vi "CSS811_Main.vi"(8 "error in":errorcluster, 11 "Enum":T1) -> (0 "error out":errorcluster, 2 "CSS811CO2_ppm":u16, 3 "CSS811_VOCppb":u16)   [LabVIEW 2016]
uses:
  CSS811_StateMachine.ctl
  <vilib>/myRIO/Instrument Drivers/Onboard IO/I2C/vis/Configure.vi
  <vilib>/myRIO/Instrument Drivers/Onboard IO/I2C/vis/Write.vi
  <vilib>/myRIO/Instrument Drivers/Onboard IO/I2C/vis/Read.vi
  <vilib>/myRIO/Instrument Drivers/Onboard IO/I2C/vis/Smart Open.vi
  <vilib>/Utility/error.llb/Error Cluster From Error Code.vi
  <vilib>/myRIO/Common/Instrument Driver Framework/myRIO v1.0/I2C/vis/myRIO v1.0 Configure I2C.vi
  <vilib>/myRIO/Common/Instrument Driver Framework/myRIO v1.0/I2C/vis/myRIO v1.0 Write I2C.vi
  <vilib>/myRIO/Common/Instrument Driver Framework/myRIO v1.0/I2C/vis/myRIO v1.0 Read I2C.vi
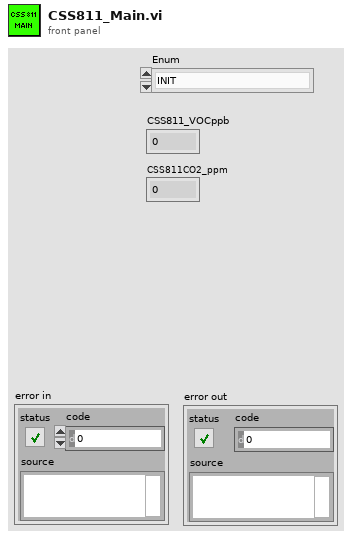
[diagram p1: front panel]
types:
  T1 = typedef "CSS811_StateMachine.ctl" = enum16{"INIT", "CHECK_STATUS", "SET_SENSOR_MODE", "SET_MEASURE_INTERVALL", "GET_SENSOR_DATA", "END", "RESET", "ERROR"}
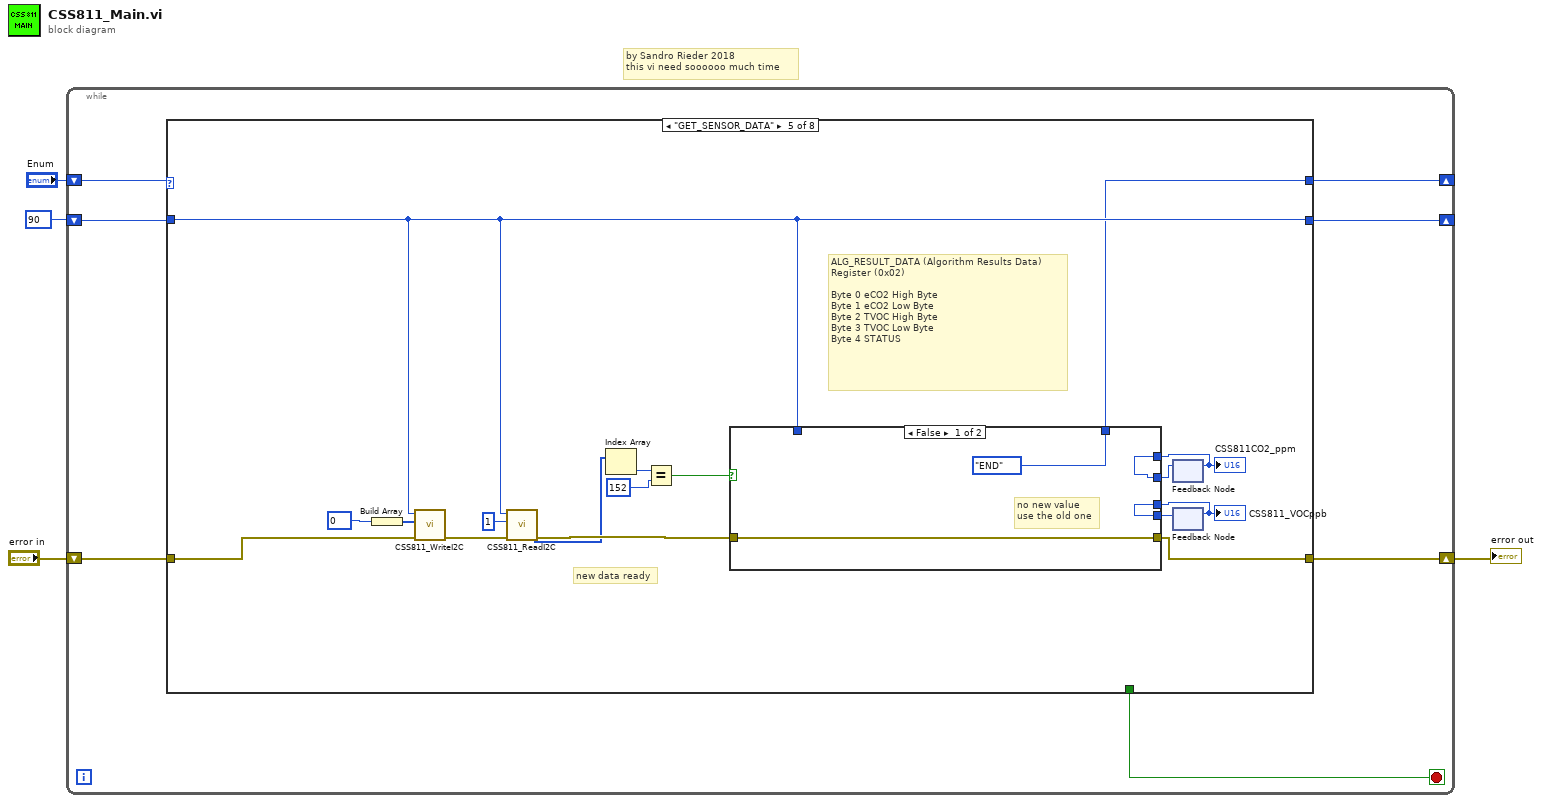
[diagram p0: block diagram]
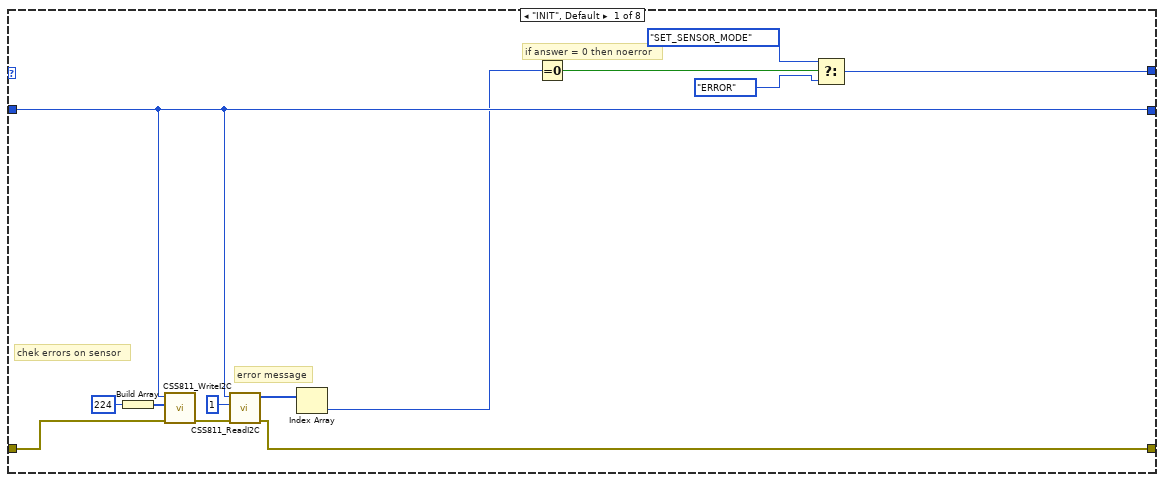
[diagram p2: hidden frame]
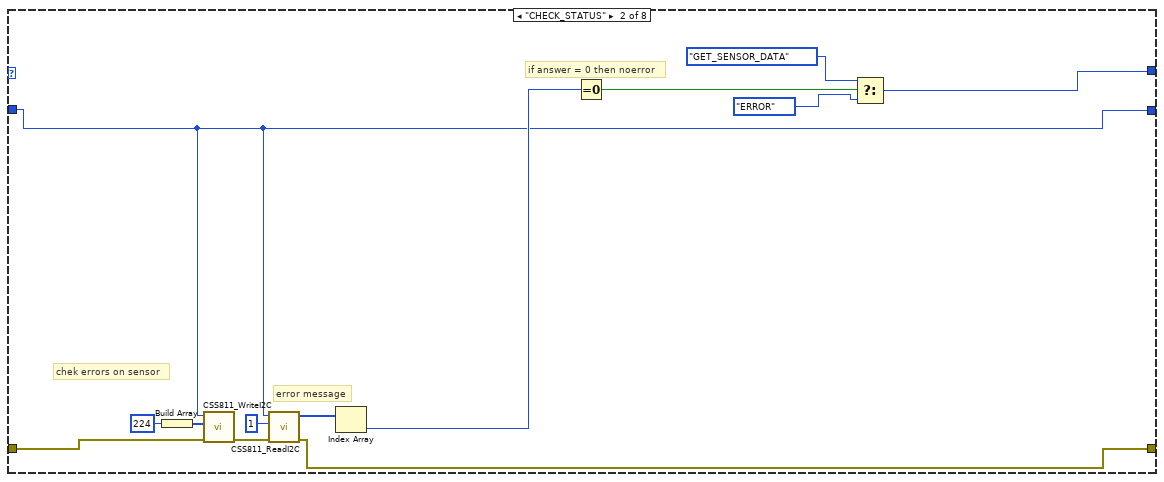
[diagram p3: hidden frame]
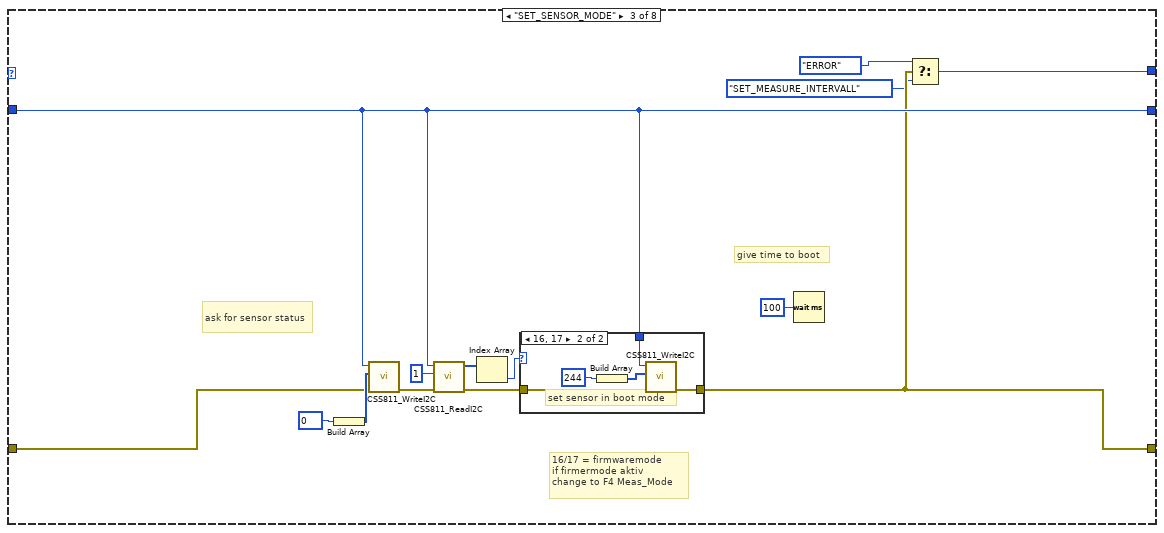
[diagram p4: hidden frame]
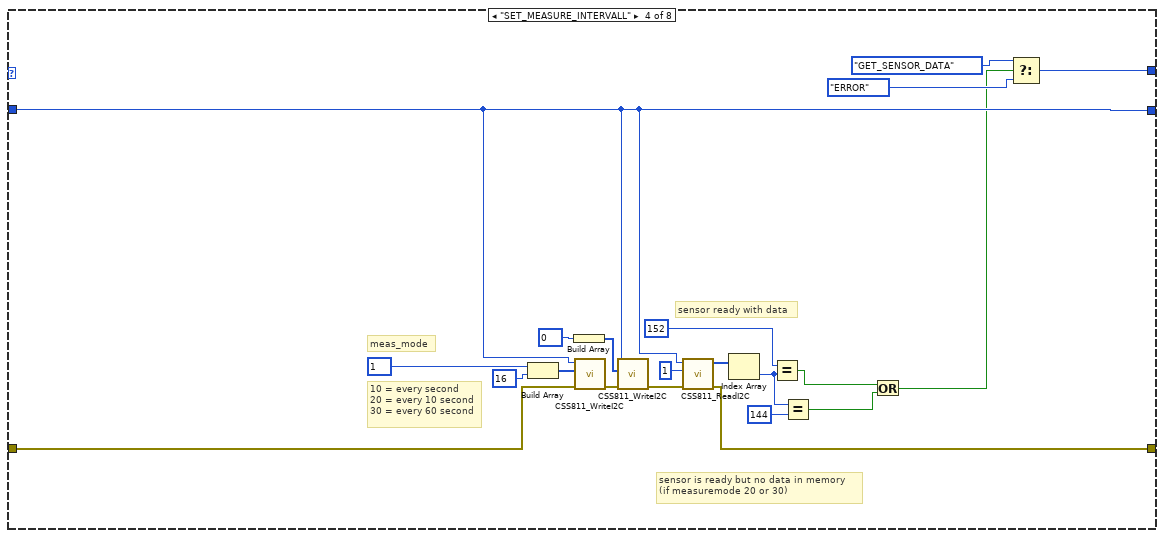
[diagram p6: hidden frame]
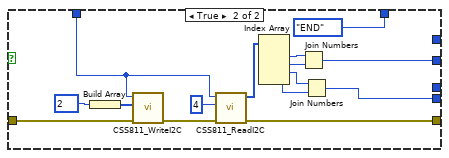
[diagram p7: hidden frame]
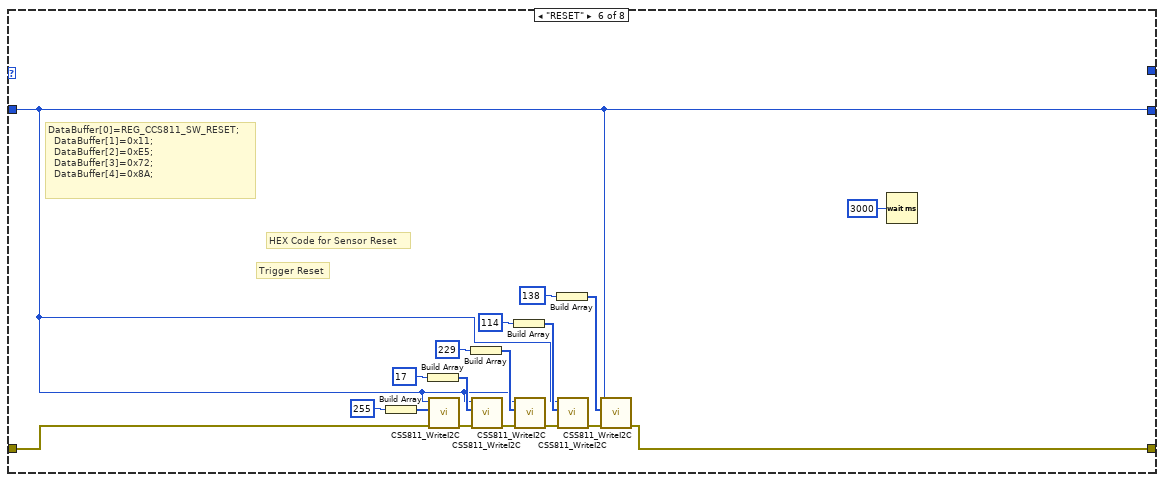
[diagram p8: hidden frame]
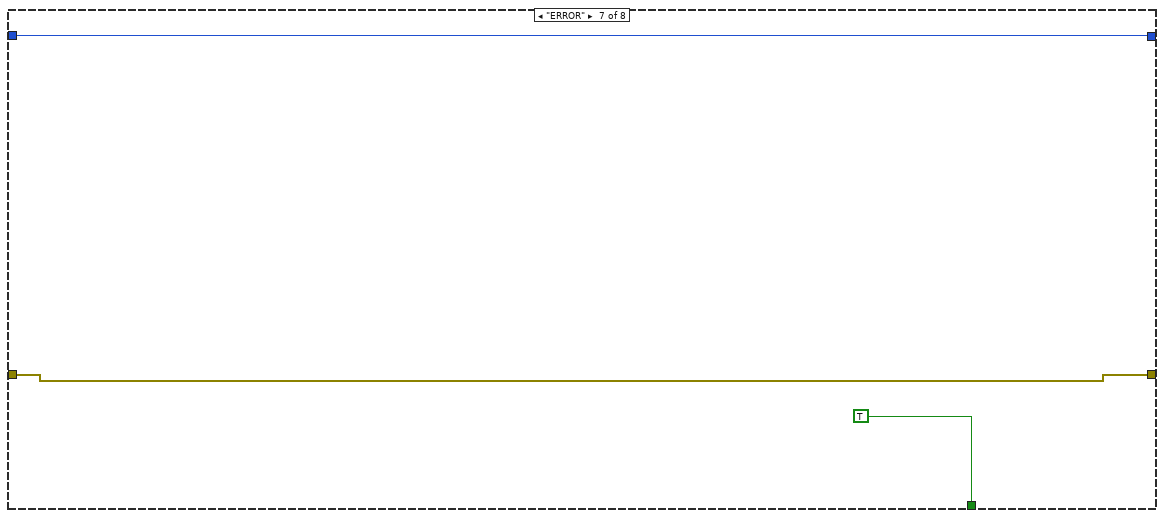
[diagram p9: hidden frame]
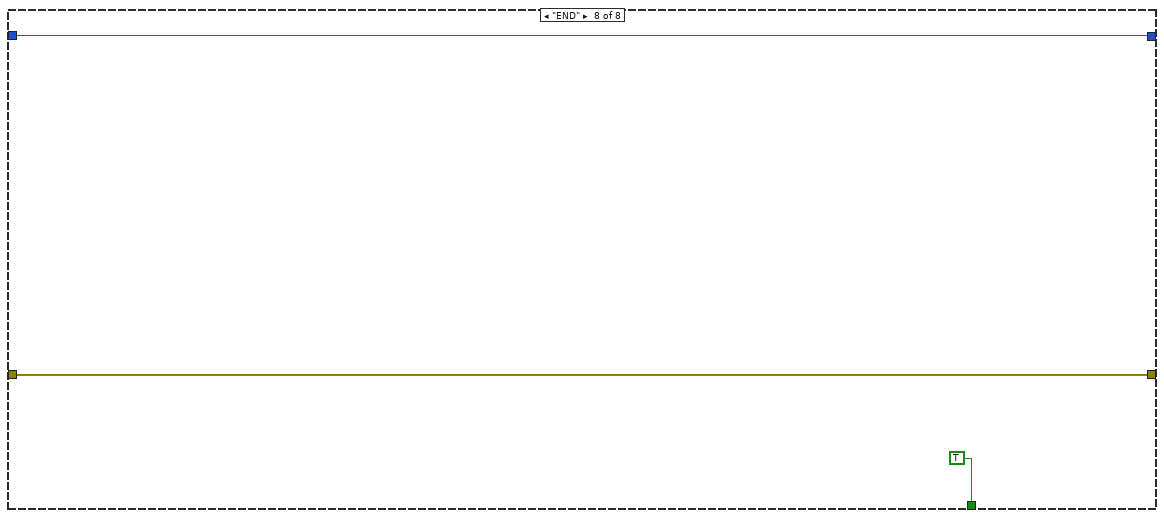
[diagram p10: hidden frame]
diagram:
  # "by Sandro Rieder 2018\nthis vi need soooooo much time"
  n1 = while {
    shift-right: [w8] -> _
    shift-left: u8 90 ("Slave Address (7-bit)") -> [w7]
    shift-right: [w10] -> w4
    shift-left: "error in" -> [w11]
    shift-right: [w6] -> _
    shift-left: "Enum" -> [w9]
    stop <- w5 stop-if-true
    n2 = case shown="\"GET_SENSOR_DATA\"" w9 {
      tunnel: w11 -> [w23 w29 w44 w75 w86 w117 w134 w137]
      tunnel: [w19 w28 w42 w67 w87 w116 w134 w137] -> w10
      tunnel: [w18 w26 w43 w66 w84 w115 w135 w138] -> w8
      tunnel: w7 -> [w18 w26 w43 w66 w84 w115 w135 w138]
      tunnel: [w12 w27 w41 w63 w83 _ _ _] -> w6
      tunnel: [_ _ _ _ _ _ TRUE TRUE] -> w5
      frame "INIT", Default {
        # "chek errors on sensor"
        # "if answer = 0 then noerror"
        # "error message"
        n3 = Build Array(u8 224) -> (w24:u8[])
        n4 = call "CSS811_WriteI2C.vi"("error in (no error)"=w23, "Bytes to Write"=w24, "Slave Address (7-bit)"=w18) -> ("error out"=w20:errorcluster)  [unwired: 6 in]
        n5 = call "CSS811_ReadI2C.vi"("error in (no error)"=w20, "Byte Count"=u32 1, "Slave Address (7-bit)"=w18) -> ("error out"=w19:errorcluster, "Bytes Read"=w17:u8[])  [unwired: 5 in]
        n6 = Index Array(array=w17) -> (element=w16:u8)  [unwired: 1 in]
        n7 = Equal To 0?(x=w16) -> (x = 0?=w15:bool)
        n8 = Select(t=CSS811_StateMachine."SET_SENSOR_MODE", s=w15, f=CSS811_StateMachine."ERROR") -> (s? t:f=w12:T1)
      }
      frame "CHECK_STATUS" {
        # "chek errors on sensor"
        # "if answer = 0 then noerror"
        # "error message"
        n9 = Build Array(u8 224) -> (w37:u8[])
        n10 = call "CSS811_WriteI2C.vi"("error in (no error)"=w29, "Bytes to Write"=w37, "Slave Address (7-bit)"=w26) -> ("error out"=w34:errorcluster)  [unwired: 6 in]
        n11 = call "CSS811_ReadI2C.vi"("error in (no error)"=w34, "Byte Count"=u32 1, "Slave Address (7-bit)"=w26) -> ("error out"=w28:errorcluster, "Bytes Read"=w33:u8[])  [unwired: 5 in]
        n12 = Index Array(array=w33) -> (element=w32:u8)  [unwired: 1 in]
        n13 = Equal To 0?(x=w32) -> (x = 0?=w31:bool)
        n14 = Select(t=CSS811_StateMachine."GET_SENSOR_DATA", s=w31, f=CSS811_StateMachine."ERROR") -> (s? t:f=w27:T1)
      }
      frame "SET_SENSOR_MODE" {
        # "give time to boot"
        # "ask for sensor status"
        # "16/17 = firmwaremode\nif firmermode aktiv\nchange to F4 Meas_Mode"
        n15 = Build Array(u8 0) -> (w46:u8[])
        n16 = call "CSS811_WriteI2C.vi"("error in (no error)"=w44, "Bytes to Write"=w46, "Slave Address (7-bit)"=w43) -> ("error out"=w47:errorcluster)  [unwired: 6 in]
        n17 = call "CSS811_ReadI2C.vi"("error in (no error)"=w47, "Byte Count"=u32 1, "Slave Address (7-bit)"=w43) -> ("error out"=w48:errorcluster, "Bytes Read"=w49:u8[])  [unwired: 5 in]
        n18 = Index Array(array=w49) -> (element=w50:u8)  [unwired: 1 in]
        n19 = case shown="16, 17" w50 {
          tunnel: [w52 w55] -> w42
          tunnel: w48 -> [w52 w54]
          tunnel: w43 -> [_ w53]
          frame 144, Default {
            # "sensor is running"
          }
          frame 16, 17 {
            # "set sensor in boot mode"
            n20 = Build Array(u8 244) -> (w56:u8[])
            n21 = call "CSS811_WriteI2C.vi"("error in (no error)"=w54, "Bytes to Write"=w56, "Slave Address (7-bit)"=w53) -> ("error out"=w55:errorcluster)  [unwired: 6 in]
          }
        }
        n22 = Wait (ms)(milliseconds to wait=u32 100) -> ()  [unwired: 1 out]
        n23 = Select(t=CSS811_StateMachine."ERROR", s=w42, f=CSS811_StateMachine."SET_MEASURE_INTERVALL") -> (s? t:f=w41:T1)
      }
      frame "SET_MEASURE_INTERVALL" {
        # "sensor is ready but no data in memory\n(if measuremode 20 or 30)"
        # "sensor ready with data"
        # "10 = every second\n20 = every 10 second\n30 = every 60 second"
        # "meas_mode"
        n24 = Build Array(u8 1, u8 16) -> (w77:u8[])
        n25 = Build Array(u8 0) -> (w72:u8[])
        n26 = call "CSS811_WriteI2C.vi"("error in (no error)"=w75, "Bytes to Write"=w77, "Slave Address (7-bit)"=w66) -> ("error out"=w68:errorcluster)  [unwired: 6 in]
        n27 = call "CSS811_WriteI2C.vi"("error in (no error)"=w68, "Bytes to Write"=w72, "Slave Address (7-bit)"=w66) -> ("error out"=w74:errorcluster)  [unwired: 6 in]
        n28 = call "CSS811_ReadI2C.vi"("error in (no error)"=w74, "Byte Count"=u32 1, "Slave Address (7-bit)"=w66) -> ("error out"=w67:errorcluster, "Bytes Read"=w70:u8[])  [unwired: 5 in]
        n29 = Index Array(array=w70) -> (element=w61:u8)  [unwired: 1 in]
        n30 = Equal?(x=u8 152, y=w61) -> (x = y?=w62:bool)
        n31 = Equal?(x=w61, y=u8 144) -> (x = y?=w59:bool)
        n32 = Or(x=w62, y=w59) -> (x .or. y?=w58:bool)
        n33 = Select(t=CSS811_StateMachine."GET_SENSOR_DATA", s=w58, f=CSS811_StateMachine."ERROR") -> (s? t:f=w63:T1)
      }
      frame "GET_SENSOR_DATA" {
        # "new data ready"
        # "ALG_RESULT_DATA (Algorithm Results Data)\nRegister (0x02)\n\nByte 0 eCO2 High Byte\nByte 1 eCO2 Low Byte\nByte 2 TVOC High Byte\nByte 3 TVOC Low Byte\nByte 4 STATUS"
        n34 = Build Array(u8 0) -> (w93:u8[])
        n35 = call "CSS811_WriteI2C.vi"("error in (no error)"=w86, "Bytes to Write"=w93, "Slave Address (7-bit)"=w84) -> ("error out"=w91:errorcluster)  [unwired: 6 in]
        n36 = call "CSS811_ReadI2C.vi"("error in (no error)"=w91, "Byte Count"=u32 1, "Slave Address (7-bit)"=w84) -> ("error out"=w95:errorcluster, "Bytes Read"=w90:u8[])  [unwired: 5 in]
        n37 = Index Array(array=w90) -> (element=w89:u8)  [unwired: 1 in]
        n38 = Equal?(x=w89, y=u8 152) -> (x = y?=w88:bool)
        n39 = feedback #1() -> (w81:u16)  [unwired: 1 in]
        "CSS811CO2_ppm" <- w81
        n40 = feedback #2() -> (w79:u16)  [unwired: 1 in]
        "CSS811_VOCppb" <- w79
        n41 = case shown="False" w88 {
          tunnel: w95 -> [w99 w108]
          tunnel: [w99 w106] -> w87
          tunnel: w84 -> [_ w103]
          tunnel: [CSS811_StateMachine."END" CSS811_StateMachine."END"] -> w83
          tunnel: [w96 w101] -> w80
          tunnel: [w97 w100] -> w82
          tunnel: w81 -> [w97 _]
          tunnel: w79 -> [w96 _]
          frame False {
            # "no new value \nuse the old one"
          }
          frame True {
            n42 = Build Array(u8 2) -> (w109:u8[])
            n43 = call "CSS811_WriteI2C.vi"("error in (no error)"=w108, "Bytes to Write"=w109, "Slave Address (7-bit)"=w103) -> ("error out"=w107:errorcluster)  [unwired: 6 in]
            n44 = call "CSS811_ReadI2C.vi"("error in (no error)"=w107, "Byte Count"=u32 4, "Slave Address (7-bit)"=w103) -> ("error out"=w106:errorcluster, "Bytes Read"=w111:u8[])  [unwired: 5 in]
            n45 = Index Array(array=w111) -> (element #1=w114:u8, element #2=w113:u8, element #3=w105:u8, element #4=w104:u8)  [unwired: 4 in]
            n46 = Join Numbers(hi=w114, lo=w113) -> ((hi.lo)=w100:u16)
            n47 = Join Numbers(hi=w105, lo=w104) -> ((hi.lo)=w101:u16)
          }
        }
        n48 = feedback-in #1(w82) -> ()
        n49 = feedback-in #2(w80) -> ()
      }
      frame "RESET" {
        # "DataBuffer[0]=REG_CCS811_SW_RESET;\n  DataBuffer[1]=0x11;\n  DataBuffer[2]=0xE5;\n  DataBuffer[3]=0x72;\n  DataBuffer[4]=0x8A;"
        # "Trigger Reset"
        # "HEX Code for Sensor Reset"
        n50 = Build Array(u8 255) -> (w128:u8[])
        n51 = Build Array(u8 17) -> (w127:u8[])
        n52 = call "CSS811_WriteI2C.vi"("error in (no error)"=w117, "Bytes to Write"=w128, "Slave Address (7-bit)"=w115) -> ("error out"=w125:errorcluster)  [unwired: 6 in]
        n53 = Build Array(u8 229) -> (w126:u8[])
        n54 = call "CSS811_WriteI2C.vi"("error in (no error)"=w125, "Bytes to Write"=w127, "Slave Address (7-bit)"=w115) -> ("error out"=w124:errorcluster)  [unwired: 6 in]
        n55 = Build Array(u8 114) -> (w122:u8[])
        n56 = call "CSS811_WriteI2C.vi"("error in (no error)"=w124, "Bytes to Write"=w126, "Slave Address (7-bit)"=w115) -> ("error out"=w123:errorcluster)  [unwired: 6 in]
        n57 = Build Array(u8 138) -> (w119:u8[])
        n58 = call "CSS811_WriteI2C.vi"("error in (no error)"=w123, "Bytes to Write"=w122, "Slave Address (7-bit)"=w115) -> ("error out"=w121:errorcluster)  [unwired: 6 in]
        n59 = call "CSS811_WriteI2C.vi"("error in (no error)"=w121, "Bytes to Write"=w119, "Slave Address (7-bit)"=w115) -> ("error out"=w116:errorcluster)  [unwired: 6 in]
        n60 = Wait (ms)(milliseconds to wait=u32 3000) -> ()  [unwired: 1 out]
      }
      frame "ERROR" {
      }
      frame "END" {
      }
    }
  }
  "error out" <- w4
